vi "LDT Telescope Generate Offset XML.vi"(8 "error in":errorcluster, 11 "Offsets":T1) -> (3 "XML String":string)   [LabVIEW 2022 SP3, in "LDT Telescope.lvclass"]
uses:
  LDT Telescope.lvclass
  CC cluster Telescope Offsets.ctl
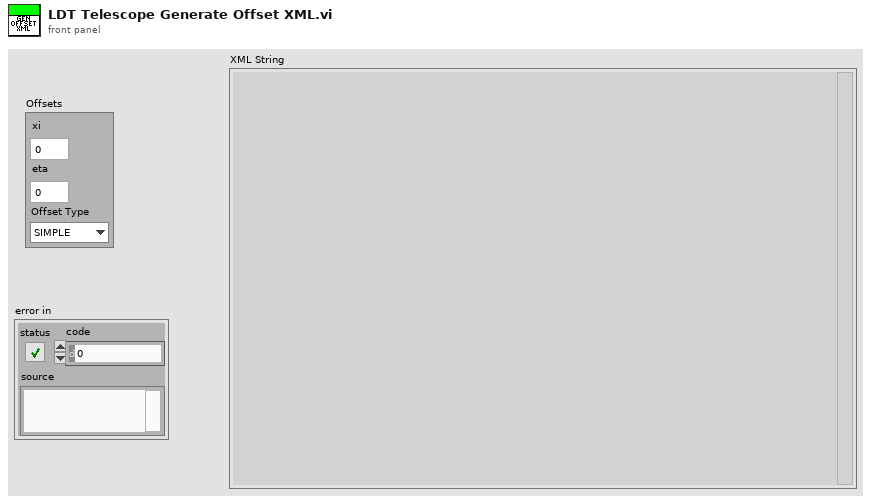
[diagram p1: front panel]
types:
  T1 = typedef "CC cluster Telescope Offsets.ctl" = cluster{"xi":dbl, "eta":dbl, "Offset Type":enum16{"SIMPLE", "TPLANE", "PA"}}
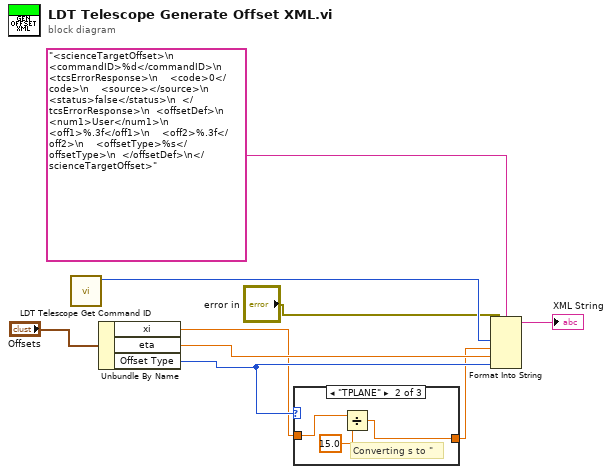
[diagram p0: block diagram]
diagram:
  n1 = call "LDT Telescope Get Command ID.vi"() -> ("Command ID"=w7:i32)  [unwired: 10 in, 1 out]
  n2 = Unbundle By Name("Offsets") -> ("xi"=w2:dbl, "eta"=w6:dbl, "Offset Type"=w3:enum16{"SIMPLE", "TPLANE", "PA"})
  n3 = case shown="\"TPLANE\"" w3 {
    tunnel: w2 -> [w10 w13 w14]
    tunnel: [w10 w11 w14] -> w1
    frame "SIMPLE", Default {
    }
    frame "TPLANE" {
      # "Converting s to \""
      n4 = Divide(x=w13, y=15.0) -> (x/y=w11:dbl)
    }
    frame "PA" {
    }
  }
  n5 = Format Into String(format string="<scienceTargetOffset>\n  <commandID>%d</commandID>\n  <tcsErrorResponse>\n    <code>0</code>\n    <source></source>\n    <status>false</status>\n  </tcsErrorResponse>\n  <offsetDef>\n    <num1>User</num1>\n    <off1>%.3f</off1>\n    <off2>%.3f</off2>\n    <offsetType>%s</offsetType>\n  </offsetDef>\n</scienceTargetOffset>", error in="error in", w7, w1, w6, w3) -> (resulting string=→"XML String":string)  [unwired: 1 in, 1 out]
